vi "hw3-5 topVI.vi"() -> ()   [LabVIEW 2014]
panel:
  out "Waveform Chart":u32(graph)=366
  in  "Stop program":bool
  out "reaction time":u32
  in  "Stop timer":bool
  out "LED":bool
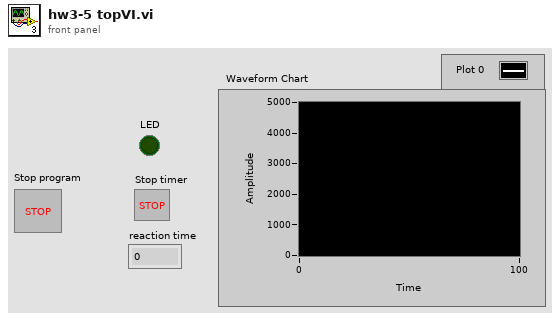
[diagram p1: front panel]
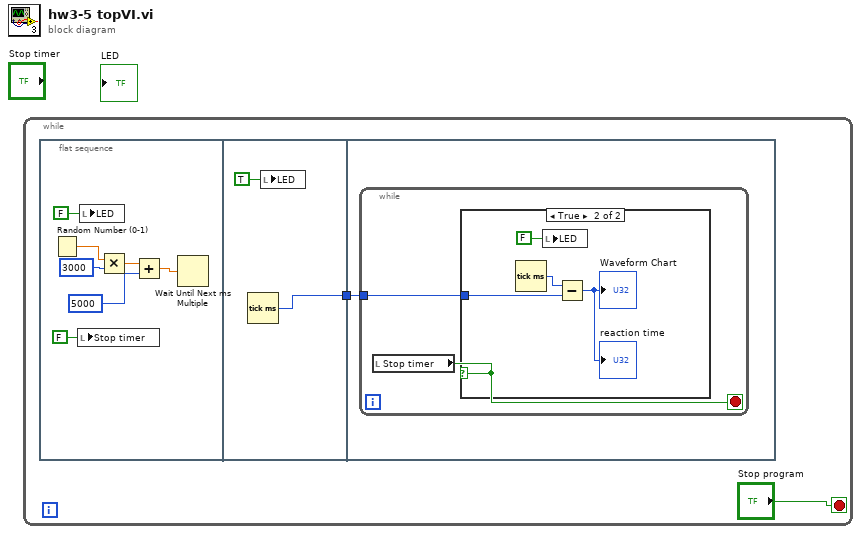
[diagram p0: block diagram]
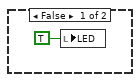
[diagram p2: hidden frame]
diagram:
  n1 = while {
    stop <- "Stop program" stop-if-true
    n2 = flat-sequence {
      tunnel: [w10] -> w2
      tunnel: w2 -> [w12]
      frame #0 {
        n3 = Random Number (0-1)() -> (number: 0 to 1=w9:dbl)
        n4 = local write "Stop timer"(FALSE) -> ()
        n5 = local write "LED"(FALSE) -> ()
        n6 = Multiply(x=w9, y=3000) -> (x*y=w8:dbl)
        n7 = Add(x=w8, y=5000) -> (x+y=w5:dbl)
        n8 = Wait Until Next ms Multiple(millisecond multiple=w5) -> ()  [unwired: 1 out]
      }
      frame #1 {
        n9 = Tick Count (ms)() -> (millisecond timer value=w10:u32)
        n10 = local write "LED"(TRUE) -> ()
      }
      frame #2 {
        n11 = while {
          tunnel: w12 -> [w13]
          stop <- w14 stop-if-true
          n12 = local read "Stop timer"() -> (w14:bool)
          n13 = case shown="True" w14 {
            tunnel: w13 -> [_ w17]
            frame False {
              n14 = local write "LED"(TRUE) -> ()
            }
            frame True {
              n15 = Tick Count (ms)() -> (millisecond timer value=w18:u32)
              n16 = local write "LED"(FALSE) -> ()
              n17 = Subtract(x=w18, y=w17) -> (x-y=→"reaction time" →"Waveform Chart":u32)
            }
          }
        }
      }
    }
  }
